vi "ClearDAQData.vi"(0 "reference in":refnum<class "DAQ_Base.lvclass">, 5 "error in (no error)":errorcluster) -> (14 "reference out":refnum<class "DAQ_Base.lvclass">, 19 "error out":errorcluster)   [LabVIEW 2020, in "DAQ.lvlib" / "DAQ_Base.lvclass"]
uses:
  DAQ_Base.lvclass
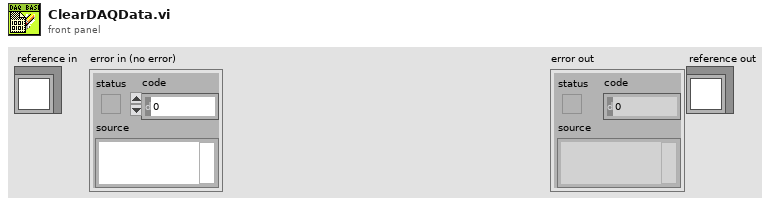
[diagram p1: front panel]
types:
  T1 = cluster{"DataCollectArry":dbl[][], "Update":bool}
  T2 = typedef "DAQ.lvlib/DAQ_Base.lvclass/DataCollector.ctl" = cluster{"DataCollectArry":dbl[][], "Update":bool}
  T3 = cluster{"CollectDataQueue":refnum<queue>, "ArryDataCollectorChannel":T2[], "RealTimeValues":dbl[]}
  T4 = cluster{"DataCollectArry":dbl[][], "Update":bool}[]
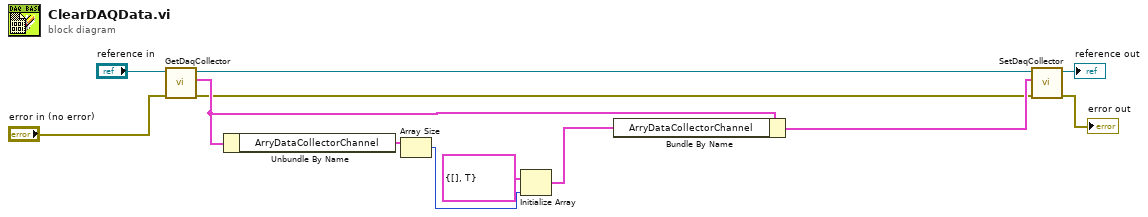
[diagram p0: block diagram]
diagram:
  n1 = call-dynamic "GetDaqCollector.vi"("error in (no error)"="error in (no error)", "reference in"="reference in") -> ("error out"=w5:errorcluster, "DaqCollector"=w7:T3, "reference out"=w12:refnum<class "DAQ_Base.lvclass">)  [unwired: 7 in]
  n2 = Unbundle By Name(w7) -> ("ArryDataCollectorChannel"=w8:T2[])
  n3 = Array Size(array=w8) -> (size(s)=w10:i32)
  n4 = Initialize Array(T1 {"DataCollectArry"=[], "Update"=TRUE} ("DataCollectorChannel"), w10) -> (w9:T4)
  n5 = Bundle By Name(cluster=w7, "ArryDataCollectorChannel"=w9) -> (w6:T3)
  n6 = call-dynamic "SetDaqCollector.vi"("error in (no error)"=w5, "DaqCollector"=w6, "reference in"=w12) -> ("error out"=→"error out":errorcluster, "reference out"=→"reference out":refnum<class "DAQ_Base.lvclass">)  [unwired: 7 in]
